vi "Main_PID.vi"() -> ()   [LabVIEW 2021]
doc: "This template is for the Queued Message Handler design pattern.\n\nThe Event Handling Loop generates messages based on user interface actions.\n\nThe Message Handling Loop processes messages generated by the Event Handling Loop, or by other messages. The messages are string values, so new messages can be added easily to the Message Cases case structure in the Message Handling Loop. Each message cluster can also provide an optional value for Message Data, which is a variant that can be converted to whatever message-specific data is required."
uses:
  Controls/UI Data.ctl
  support/Message Queue/Message Queue.lvlib
  support/User Event - Stop/User Event - Stop.lvlib
  support/Message Queue/Enqueue Message (Single).vi
  Controls/Status Lights.ctl
  Controls/Timer Actions.ctl
  <vilib>/ErrorRing/Error Ring.xnode
  <vilib>/Utility/error.llb/Error Cluster From Error Code.vi
panel:
  in  "Horizontal Slide Switch":bool
  out "Target Speed":dbl format="%.2f"
  in  "Target Pressure (Bar)":dbl
  in  "Start PID Control":bool
  out "Sampling Active":bool=TRUE
  out "Pressure":dbl(knob) scale=0.0..10.0
  out "Pressure (Bar)":dbl
  out "Sampling State":string
  in  "Start Pressure Logging":bool
  out "Speed Indicator":dbl
  in  "Release Brake":bool
  out "Status":T1
  in  "Speed (v)":dbl(knob) min=-5.0 max=5.0 scale=-5.0..5.0
  out "Status Message":string
  in  "Apply Brake":bool
  in  "Exit":bool
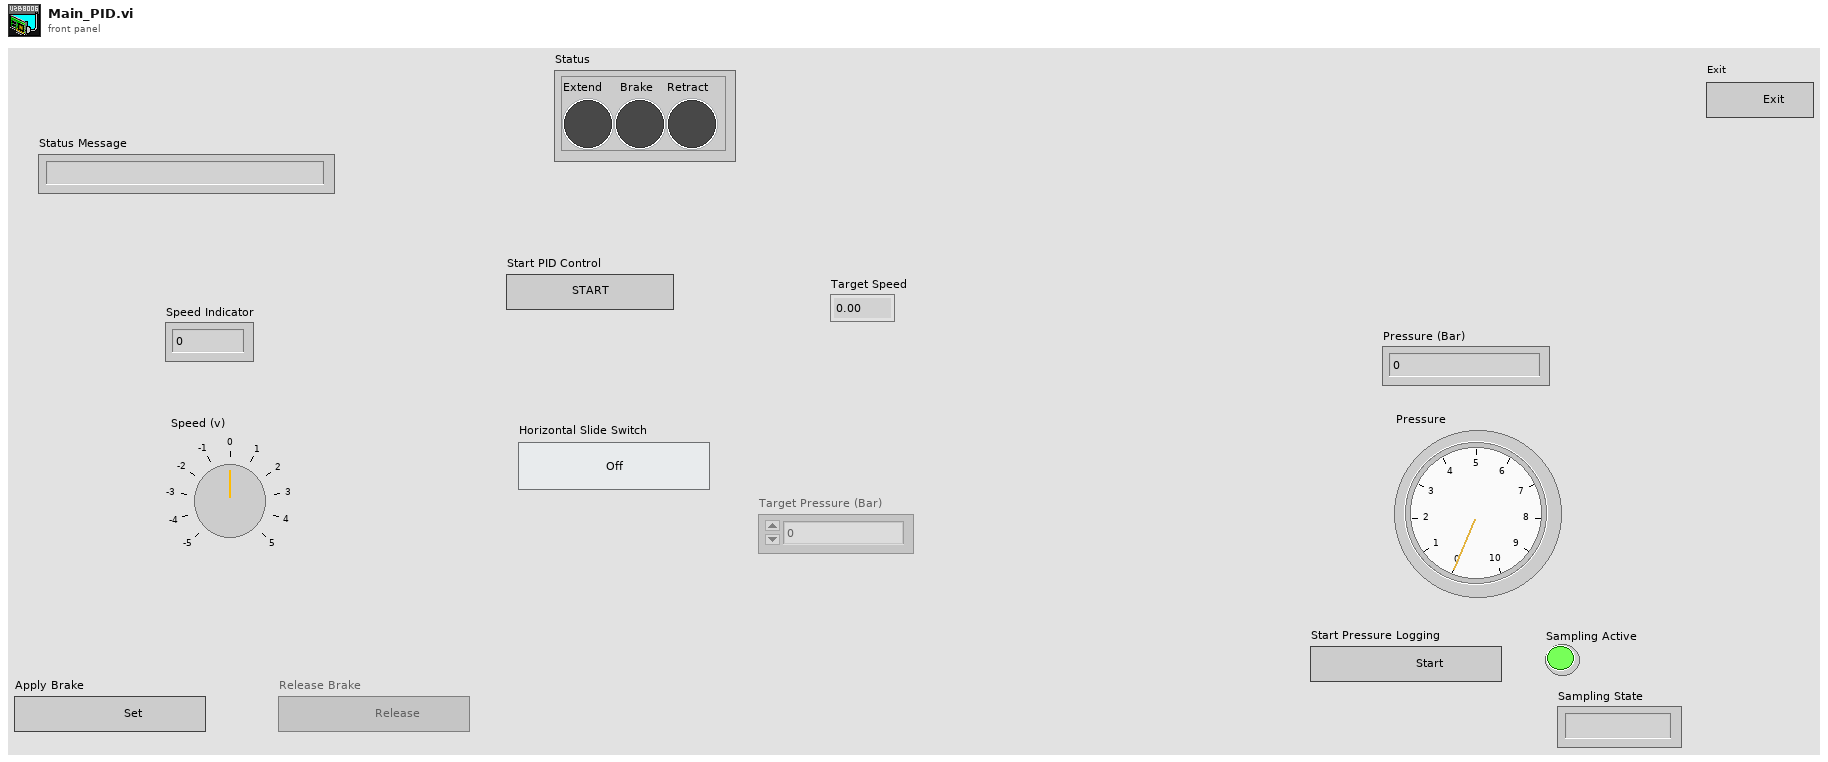
[diagram p1: front panel]
types:
  T1 = typedef "Status Lights.ctl" = cluster{"Extend":bool, "Brake":bool, "Retract":bool}
  T2 = cluster{"Apply Brake FP":enum8{"Enabled", "Disabled", "Disabled and Grayed Out"}, "Release Brake FP":enum8{"Enabled", "Disabled", "Disabled and Grayed Out"}, "Extend FP":enum8{"Enabled", "Disabled", "Disabled and Grayed Out"}, "Retract FP":enum8{"Enabled", "Disabled", "Disabled and Grayed Out"}, "Pressure Log FP":enum8{"Enabled", "Disabled", "Disabled and Grayed Out"}, "Speed FP":enum8{"Enabled", "Disabled", "Disabled and Grayed Out"}, "Target Pressure FP":enum8{"Enabled", "Disabled", "Disabled and Grayed Out"}}
  T3 = typedef "UI Data.ctl" = cluster{"Sampling State":string, "Status Message":string, "Speed":dbl, "Pressure":dbl, "Target Pressure":dbl, "Apply Brake Ref":refnum<vi>, "Release Brake Ref":refnum<vi>, "Extend Ref":refnum<vi>, "Retract Ref":refnum<vi>, "Pressure Ref":refnum<vi>, "Data Display Ref":refnum<vi>, "Exit Button Ref":refnum<vi>, "Speed Pressure Select":bool, "Status":T1}
  T4 = typedef "Message Queue.lvlib/All Message Queues.ctl" = cluster{"UI":refnum<queue>}
  T5 = typedef "DAQ Refnums.ctl" = cluster{"Direction Ref":refnum<k21>, "Brake Ref":refnum<k21>, "Speed Ref":refnum<k21>, "Pressure Ref":refnum<k21>}
  T6 = enum8{"Enabled", "Disabled", "Disabled and Grayed Out"}
  T7 = typedef "Timer Actions.ctl" = enum16{"Start Timer", "Restart Timer", "Check Timer", "Pause Timer", "Reset Timer", "Exit Timer"}
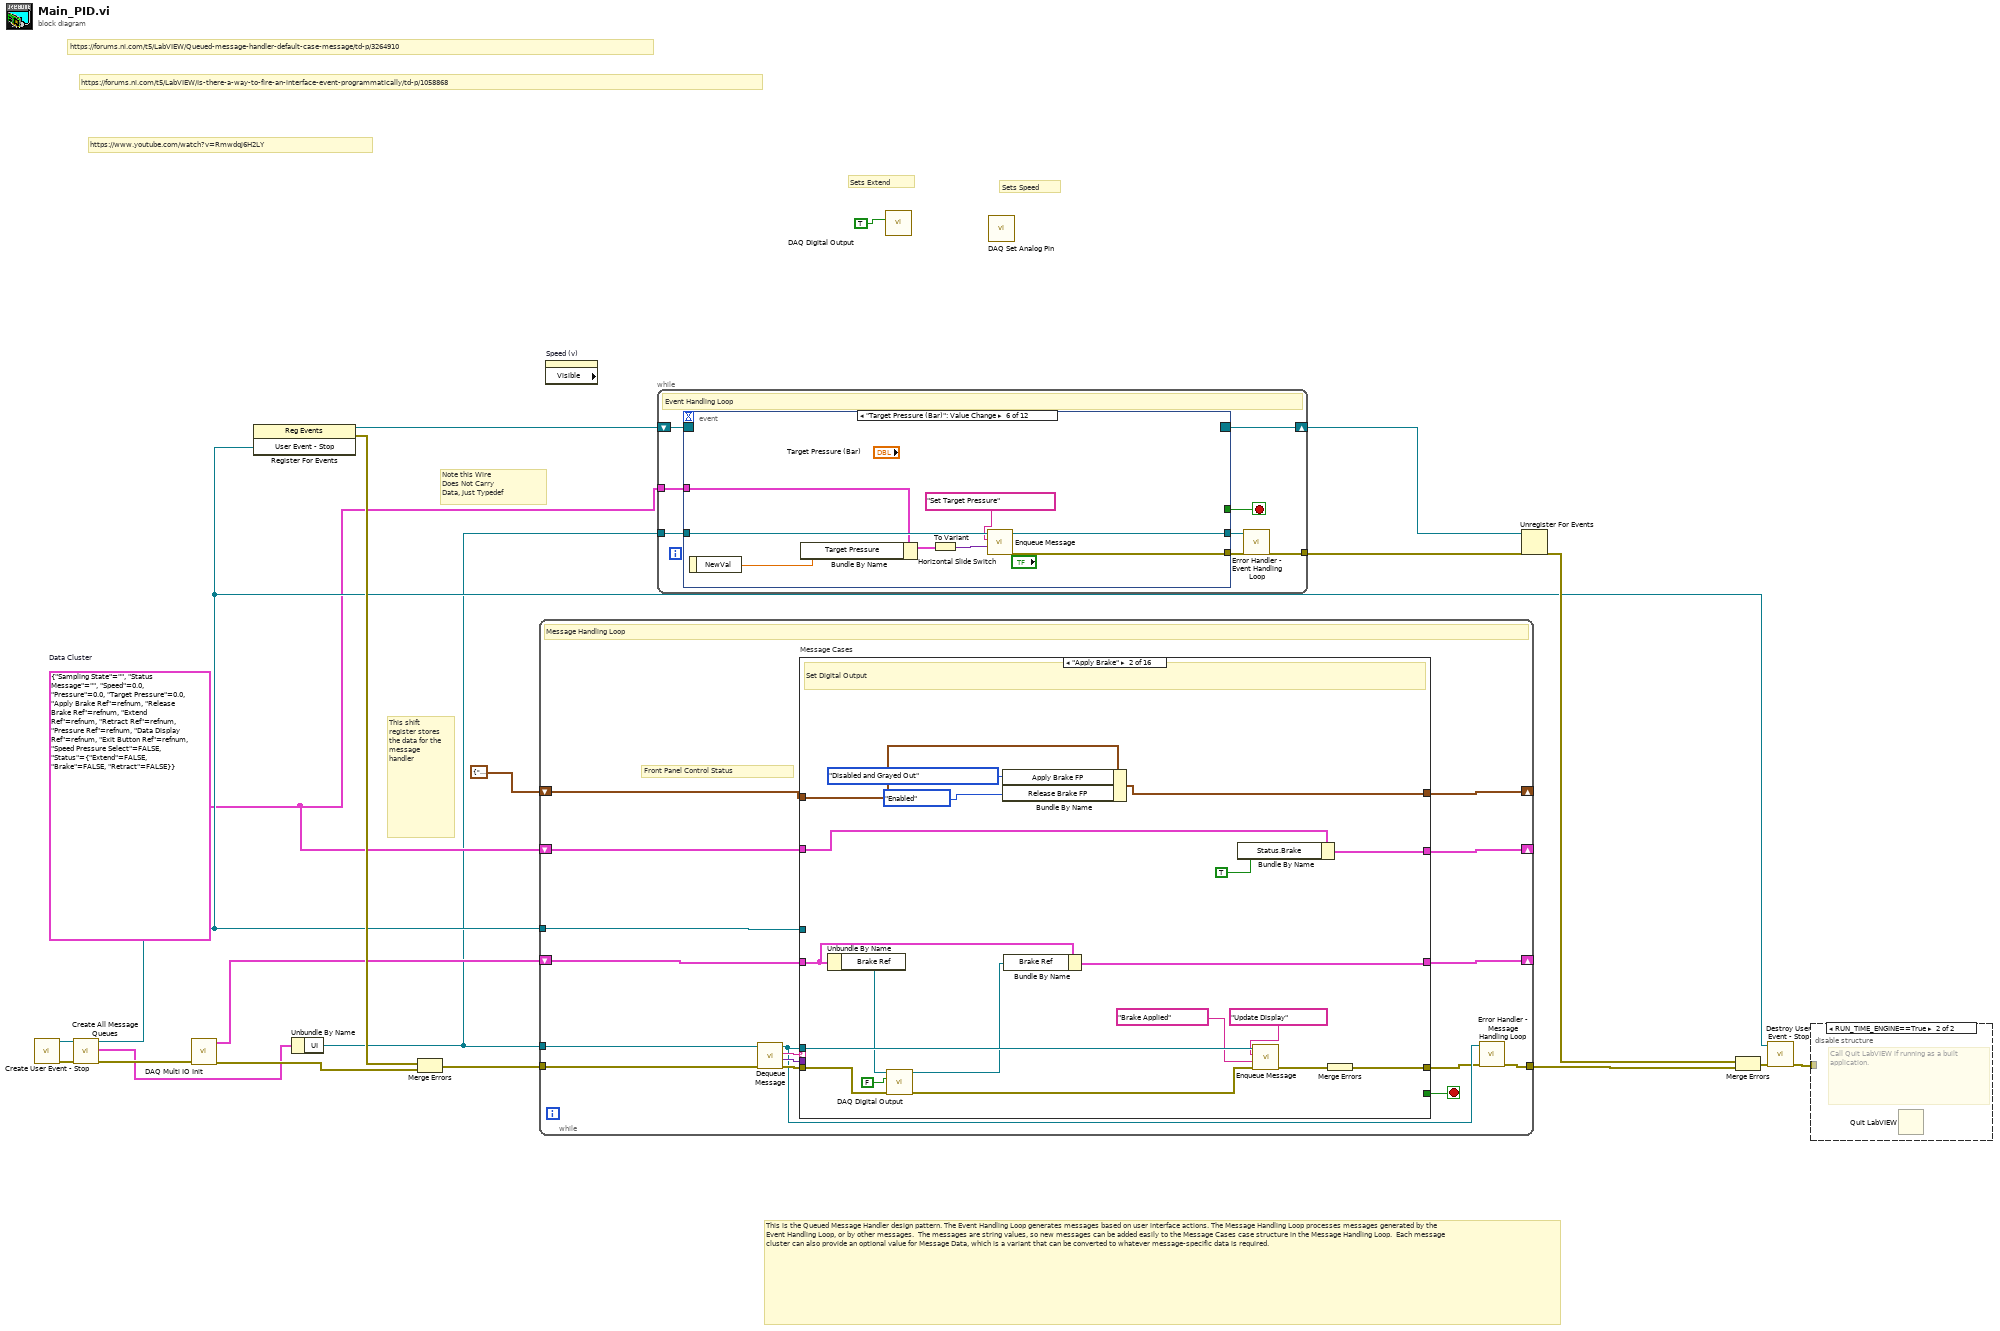
[diagram p0: block diagram]
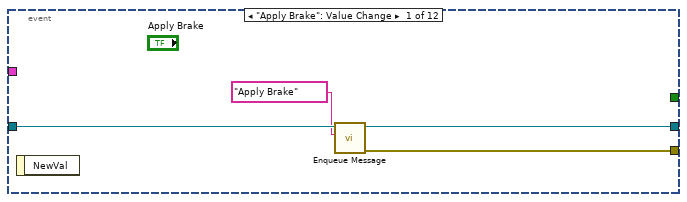
[diagram p3: hidden frame]
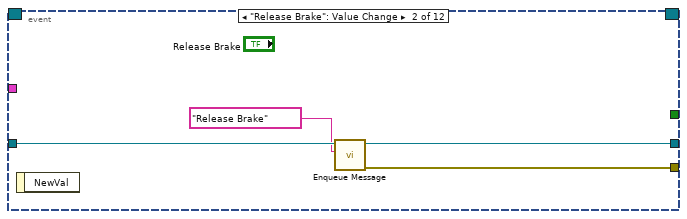
[diagram p4: hidden frame]
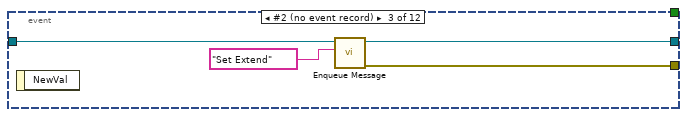
[diagram p5: hidden frame]
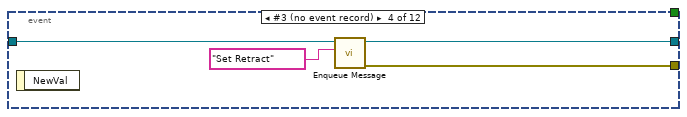
[diagram p6: hidden frame]
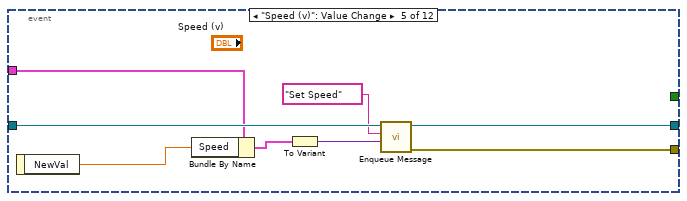
[diagram p7: hidden frame]
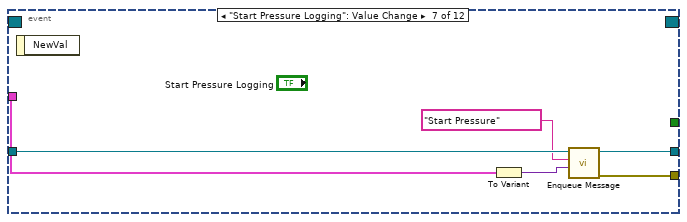
[diagram p8: hidden frame]
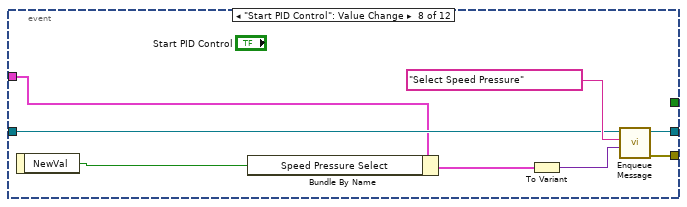
[diagram p9: hidden frame]
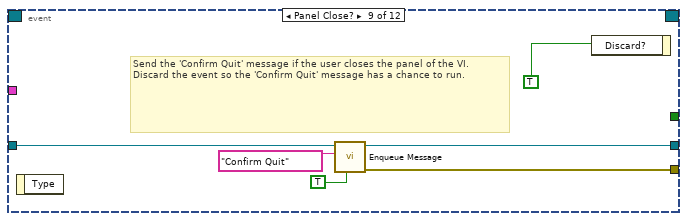
[diagram p10: hidden frame]
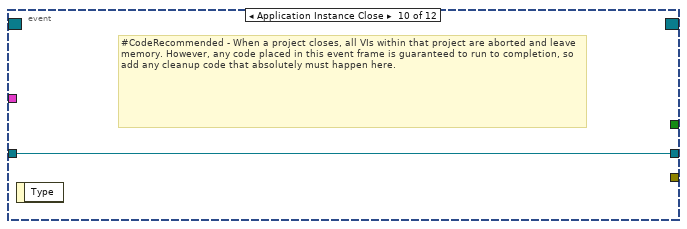
[diagram p11: hidden frame]
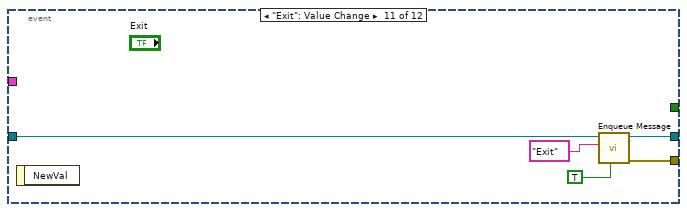
[diagram p12: hidden frame]
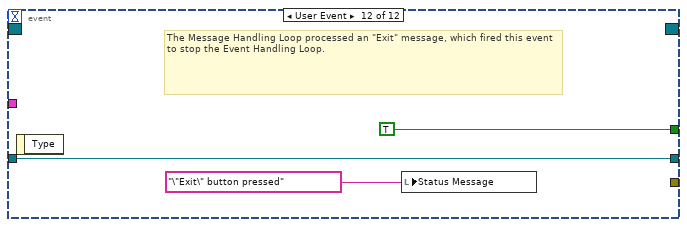
[diagram p13: hidden frame]
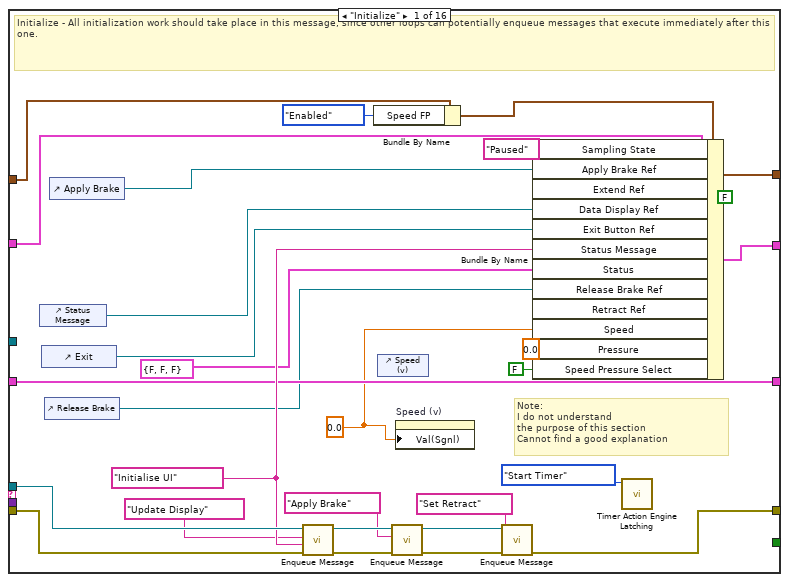
[diagram p14: hidden frame]
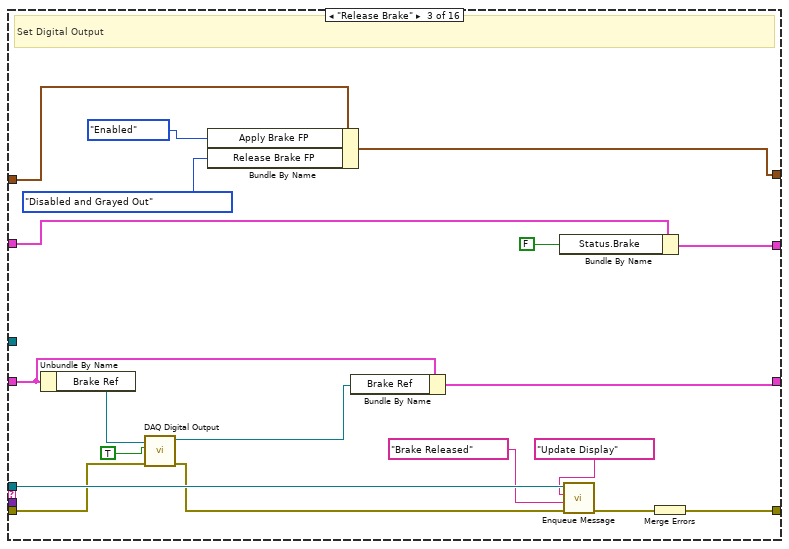
[diagram p15: hidden frame]
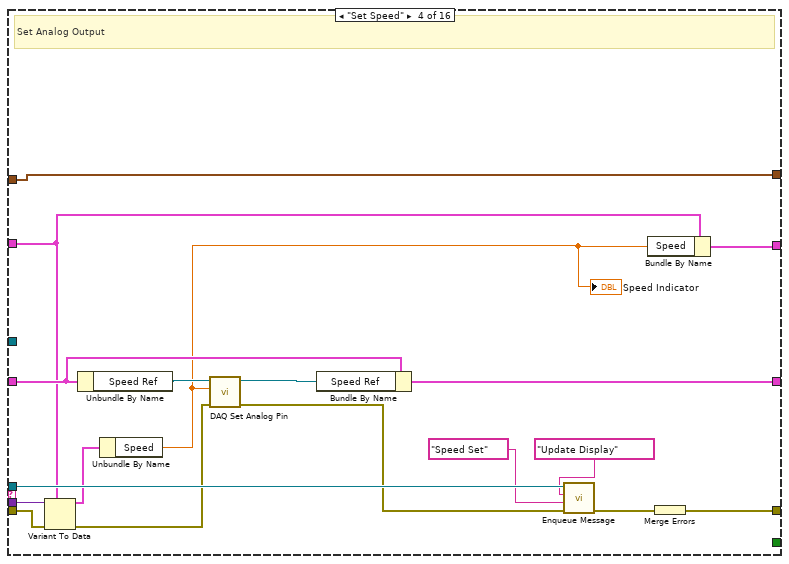
[diagram p16: hidden frame]
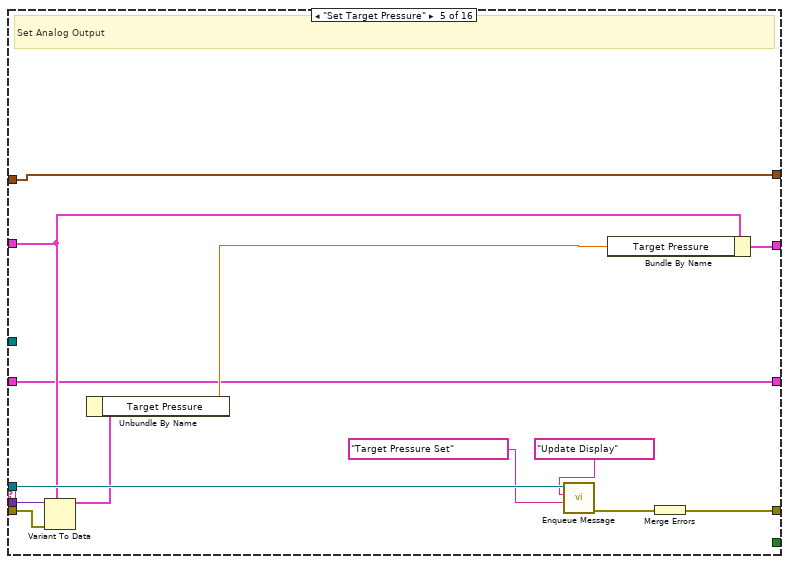
[diagram p17: hidden frame]
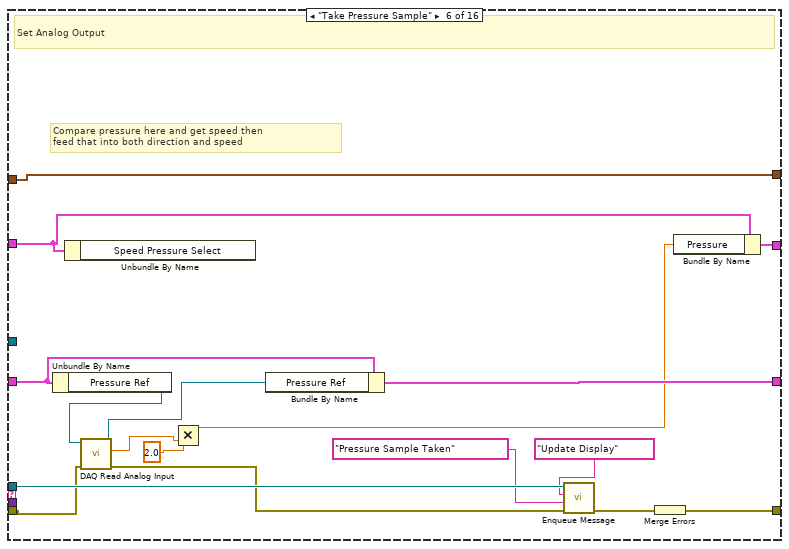
[diagram p18: hidden frame]
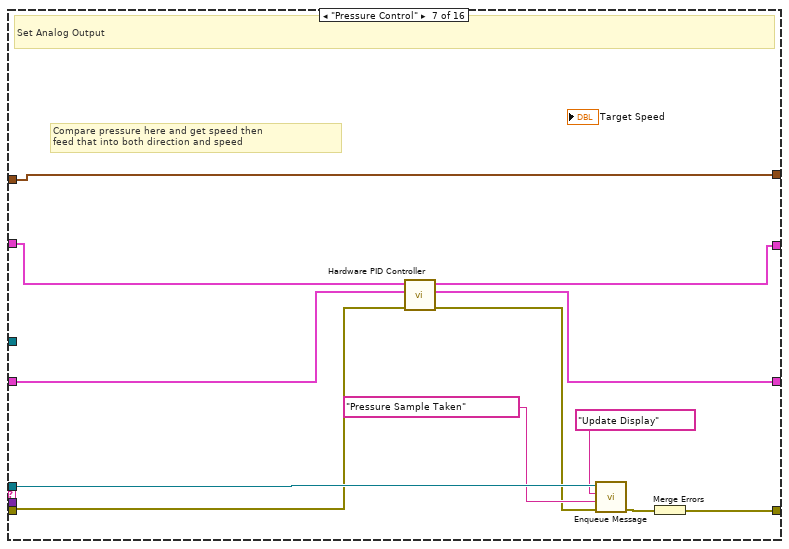
[diagram p19: hidden frame]
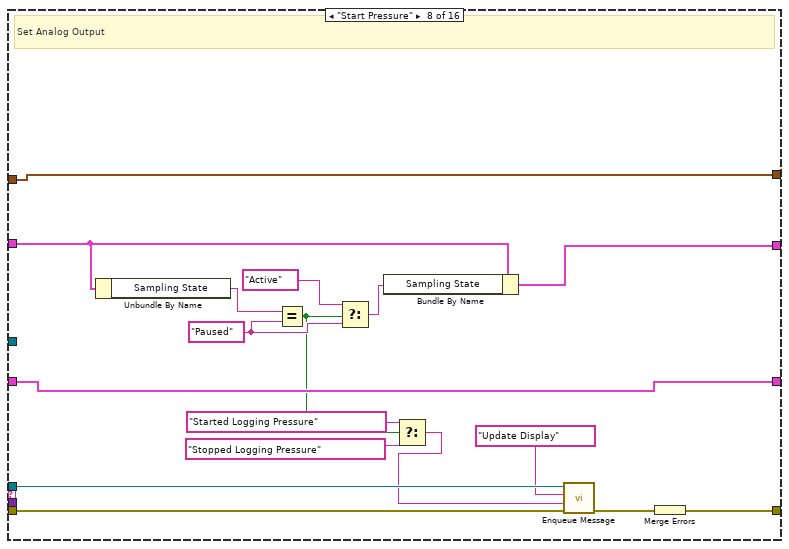
[diagram p20: hidden frame]
diagram:
  w4 = T3 {"Sampling State"="", "Status Message"="", "Speed"=0.0, "Pressure"=0.0, "Target Pressure"=0.0, "Apply Brake Ref"=refnum, "Release Brake Ref"=refnum, "Extend Ref"=refnum, "Retract Ref"=refnum, "Pressure Ref"=refnum, "Data Display Ref"=refnum, "Exit Button Ref"=refnum, "Speed Pressure Select"=FALSE, "Status"={"Extend"=FALSE, "Brake"=FALSE, "Retract"=FALSE}}  # Data Cluster
  # "Sets Speed"
  # "Sets Extend"
  # "Note this Wire\nDoes Not Carry\nData, Just Typedef"
  # "https://www.youtube.com/watch?v=Rmwdqj6H2LY"
  # "https://forums.ni.com/t5/LabVIEW/Is-there-a-way-to-fire-an-interface-event-programmatically/td-p/1058868"
  # "https://forums.ni.com/t5/LabVIEW/Queued-message-handler-default-case-message/td-p/3264910"
  # "This is the Queued Message Handler design pattern. The Event Handling Loop generates messages based on user interface actions. The Message Handling Loop processes messages generated by the Event Handling Loop, or by other messages.  The messages are string values, so new messages can be added easily to the Message Cases case structure in the Message Handling Loop.  Each message cluster can also provide an optional value for Message Data, which is a variant that can be converted to whatever message-specific data is required."
  # "This shift register stores the data for the message handler"
  n1 = call "Create User Event - Stop.vi"() -> ("error out"=w19:errorcluster, "User Event - Stop"=w8:refnum<user-event>)  [unwired: 10 in]
  n2 = call "Create All Message Queues.vi"("error in (no error)"=w19) -> ("error out"=w7:errorcluster, "Message Queues out"=w5:T4)  [unwired: 9 in]
  n3 = call "DAQ Multi IO Init.vi"("error in"=w7) -> ("error out"=w6:errorcluster, "DAQ Ref Cluster"=w9:T5)  [unwired: 9 in]
  n4 = register-events(w8) -> (reference out=w13:refnum<event-registration>, error out=w12:errorcluster)  [unwired: 2 in]
  n5 = Unbundle By Name(w5) -> ("UI"=w3:refnum<queue>)
  n6 = Merge Errors(w12, w6) -> (w10:errorcluster)
  n7 = while {
    tunnel: w3 -> [w29]
    shift-right: [w24] -> _
    shift-left: w4 -> [w35]
    tunnel: w8 -> [w33]
    tunnel: [w27] -> w11
    tunnel: w10 -> [w25]
    shift-right: [w22] -> _
    shift-left: w9 -> [w23]
    shift-right: [w20] -> _
    shift-left: T2 {"Apply Brake FP"=enum."Disabled and Grayed Out", "Release Brake FP"=enum."Disabled and Grayed Out", "Extend FP"=enum."Disabled and Grayed Out", "Retract FP"=enum."Disabled and Grayed Out", "Pressure Log FP"=enum."Disabled and Grayed Out", "Speed FP"=enum."Disabled and Grayed Out", "Target Pressure FP"=enum."Disabled and Grayed Out"} -> [w21]
    stop <- w34 stop-if-true
    # "Front Panel Control Status"
    # "Message Handling Loop"
    n8 = call "Dequeue Message.vi"("error in (no error)"=w25, "Message Queue"=w29) -> ("error out"=w32:errorcluster, "Message Data"=w30:variant, "Message"=w31:string, "dup Message Queue"=w28:refnum<queue>)  [unwired: 6 in]
    n9 = case "Message Cases" shown="\"Apply Brake\"" w31 {
      selector: w31 -> [_ _ _ _ _ _ _ _ _ _ _ _ _ _ _ w292]
      tunnel: w28 -> [w58 w79 w98 w116 w129 w146 w158 w175 w182 w205 _ w228 _ w243 w289 _]
      tunnel: w32 -> [w62 w77 w96 w107 w125 w135 w151 w167 w184 w209 w223 w232 w237 w247 w284 _]
      tunnel: [w45 w81 w100 w118 w131 w148 w160 w177 w183 w214 w217 w230 w235 w250 w286 w293] -> w26
      tunnel: w35 -> [w51 w71 w86 w104 w123 w133 w149 w168 w181 w197 w222 w231 w236 w241 w288 w294]
      tunnel: [w61 w74 w93 w103 w122 w141 w153 w170 w181 w197 w222 w231 w236 w240 w288 w294] -> w24
      tunnel: [_ _ _ _ _ _ _ _ _ _ _ _ _ _ TRUE _] -> w34
      tunnel: w30 -> [_ _ _ w108 w126 _ _ _ _ w210 w221 _ _ w248 w281 _]
      tunnel: w33 -> [_ _ _ _ _ _ _ _ _ _ _ _ _ _ w285 _]
      tunnel: w23 -> [w54 w69 w88 w113 w119 w143 w155 w171 w185 w212 w216 w225 w234 w249 w273 w291]
      tunnel: [w54 w68 w87 w112 w119 w142 w154 w171 w185 w212 w216 w225 w234 w249 w274 w291] -> w22
      tunnel: w21 -> [w38 w66 w85 w101 w120 w134 w150 w161 w178 w203 w215 w224 w233 w245 w267 w290]
      tunnel: [w39 w63 w82 w101 w120 w134 w150 w161 w178 w203 w215 w224 w233 w244 w267 w290] -> w20
      frame "Initialize" {
        (unwired) FALSE ("Clock Output")
        w52 = 0.0 ("Speed")
        w57 = "Initialise UI" ("Initial Message")
        # "Note:\nI do not understand\nthe purpose of this section\nCannot find a good explanation"
        # "Initialize - All initialization work should take place in this message, since other loops can potentially enqueue messages that execute immediately after this one."
        n10 = control-ref of="Status Message"() -> (w60:refnum<vi>)
        n11 = control-ref of="Exit"() -> (w59:refnum<vi>)
        n12 = control-ref of="Release Brake"() -> (w53:refnum<vi>)
        n13 = control-ref of="Apply Brake"() -> (w56:refnum<vi>)
        n14 = call-poly "Enqueue Message.vi"("error in (no error)"=w62, "Message Data"=w57, "Message"="Update Display", "Message Queue"=w58) -> ("error out"=w49:errorcluster, "dup Message Queue"=w48:refnum<queue>)  [unwired: 6 in]
        n15 = Bundle By Name(cluster=w38, "Speed FP"=T6."Enabled") -> (w39:T2)
        n16 = control-ref of="Speed (v)"() -> ()  [unwired: 1 out]
        n17 = call-poly "Enqueue Message.vi"("error in (no error)"=w49, "Message"="Apply Brake", "Message Queue"=w48) -> ("error out"=w46:errorcluster, "dup Message Queue"=w44:refnum<queue>)  [unwired: 7 in]
        n18 = property on="Speed (v)" class="Knob (strict)"("Val(Sgnl)"=w52) -> ()  [unwired: 2 in, 2 out]
        n19 = call-poly "Enqueue Message.vi"("error in (no error)"=w46, "Message"="Set Retract", "Message Queue"=w44) -> ("error out"=w45:errorcluster)  [unwired: 7 in, 1 out]
        n20 = Bundle By Name(cluster=w51, "Sampling State"="Paused", "Apply Brake Ref"=w56, "Data Display Ref"=w60, "Exit Button Ref"=w59, "Status Message"=w57, "Status"=T1 {"Extend"=FALSE, "Brake"=FALSE, "Retract"=FALSE}, "Release Brake Ref"=w53, "Speed"=w52, "Pressure"=0.0, "Speed Pressure Select"=FALSE) -> (w61:T3)  [unwired: 2 in]
        n21 = call "Timer Action Engine Latching.vi"("Action"=Timer_Actions."Start Timer") -> ()  [unwired: 7 in, 4 out]
      }
      frame "Apply Brake" {
        # "Set Digital Output"
        n22 = Unbundle By Name(w69) -> ("Brake Ref"=w70:refnum<k21>)
        n23 = call "DAQ Digital Output.vi"("error in"=w77, "data"=FALSE, "task/channels in"=w70) -> ("error out"=w76:errorcluster, "task out"=w67:refnum<k21>)  [unwired: 6 in, 1 out]
        n24 = Bundle By Name(cluster=w66, "Apply Brake FP"=T6."Disabled and Grayed Out" ("Disabled"), "Release Brake FP"=T6."Enabled" ("Disabled")) -> (w63:T2)
        n25 = Bundle By Name(cluster=w69, "Brake Ref"=w67) -> (w68:T5)
        n26 = Bundle By Name(cluster=w71, "Status.Brake"=TRUE) -> (w74:T3)
        n27 = call-poly "Enqueue Message.vi"("error in (no error)"=w76, "Message Data"="Brake Applied" ("\"Do Something\" button pressed"), "Message"="Update Display", "Message Queue"=w79) -> ("error out"=w80:errorcluster)  [unwired: 6 in, 1 out]
        n28 = Merge Errors(w80) -> (w81:errorcluster)
      }
      frame "Release Brake" {
        # "Set Digital Output"
        n29 = Unbundle By Name(w88) -> ("Brake Ref"=w90:refnum<k21>)
        n30 = call "DAQ Digital Output.vi"("error in"=w96, "data"=TRUE, "task/channels in"=w90) -> ("error out"=w95:errorcluster, "task out"=w89:refnum<k21>)  [unwired: 6 in, 1 out]
        n31 = Bundle By Name(cluster=w85, "Apply Brake FP"=T6."Enabled" ("Disabled"), "Release Brake FP"=T6."Disabled and Grayed Out" ("Disabled")) -> (w82:T2)
        n32 = Bundle By Name(cluster=w88, "Brake Ref"=w89) -> (w87:T5)
        n33 = Bundle By Name(cluster=w86, "Status.Brake"=FALSE ("Boolean")) -> (w93:T3)
        n34 = call-poly "Enqueue Message.vi"("error in (no error)"=w95, "Message Data"="Brake Released" ("\"Do Something\" button pressed"), "Message"="Update Display", "Message Queue"=w98) -> ("error out"=w99:errorcluster)  [unwired: 6 in, 1 out]
        n35 = Merge Errors(w99) -> (w100:errorcluster)
      }
      frame "Set Speed" {
        # "Set Analog Output"
        n36 = Variant To Data(error in=w107, type=w104, Variant=w108) -> (data=w105:T3, error out=w106:errorcluster)
        n37 = Unbundle By Name(w113) -> ("Speed Ref"=w111:refnum<k21>)
        n38 = Unbundle By Name(w105) -> ("Speed"=w102:dbl)
        "Speed Indicator" <- w102
        n39 = call "DAQ Set Analog Pin.vi"("error in"=w106, "Voltage"=w102, "task/channels in"=w111) -> ("error out"=w109:errorcluster, "task out"=w110:refnum<k21>)  [unwired: 6 in, 1 out]
        n40 = Bundle By Name(cluster=w113, "Speed Ref"=w110) -> (w112:T5)
        n41 = call-poly "Enqueue Message.vi"("error in (no error)"=w109, "Message Data"="Speed Set" ("\"Do Something\" button pressed"), "Message"="Update Display", "Message Queue"=w116) -> ("error out"=w117:errorcluster)  [unwired: 6 in, 1 out]
        n42 = Bundle By Name(cluster=w104, "Speed"=w102) -> (w103:T3)
        n43 = Merge Errors(w117) -> (w118:errorcluster)
      }
      frame "Set Target Pressure" {
        # "Set Analog Output"
        n44 = Variant To Data(error in=w125, type=w123, Variant=w126) -> (data=w124:T3)  [unwired: 1 out]
        n45 = Unbundle By Name(w124) -> ("Target Pressure"=w121:dbl)
        n46 = call-poly "Enqueue Message.vi"("Message Data"="Target Pressure Set" ("\"Do Something\" button pressed"), "Message"="Update Display", "Message Queue"=w129) -> ("error out"=w130:errorcluster)  [unwired: 7 in, 1 out]
        n47 = Bundle By Name(cluster=w123, "Target Pressure"=w121) -> (w122:T3)
        n48 = Merge Errors(w130) -> (w131:errorcluster)
      }
      frame "Take Pressure Sample" {
        # "Compare pressure here and get speed then \nfeed that into both direction and speed"
        # "Set Analog Output"
        n49 = Unbundle By Name(w143) -> ("Pressure Ref"=w140:refnum<k21>)
        n50 = Unbundle By Name(w133) -> ()  [unwired: 1 out]
        n51 = call "DAQ Read Analog Input.vi"("error in"=w135, "task/channels in"=w140) -> ("error out"=w139:errorcluster, "Voltage"=w137:dbl, "task out"=w138:refnum<k21>)  [unwired: 7 in]
        n52 = Multiply(x=2.0, y=w137) -> (x*y=w132:dbl)
        n53 = Bundle By Name(cluster=w143, "Pressure Ref"=w138) -> (w142:T5)
        n54 = call-poly "Enqueue Message.vi"("error in (no error)"=w139, "Message Data"="Pressure Sample Taken" ("\"Do Something\" button pressed"), "Message"="Update Display", "Message Queue"=w146) -> ("error out"=w147:errorcluster)  [unwired: 6 in, 1 out]
        n55 = Merge Errors(w147) -> (w148:errorcluster)
        n56 = Bundle By Name(cluster=w133, "Pressure"=w132) -> (w141:T3)
      }
      frame "Pressure Control" {
        # "Compare pressure here and get speed then \nfeed that into both direction and speed"
        # "Set Analog Output"
        n57 = call "Hardware PID Controller.vi"("error in (no error)"=w151, "DAQ Ref Cluster in"=w155, "State Machine Data"=w149) -> ("error out"=w152:errorcluster, "DAQ Ref Cluster out"=w154:T5, "Data Cluster out"=w153:T3)  [unwired: 6 in]
        n58 = call-poly "Enqueue Message.vi"("error in (no error)"=w152, "Message Data"="Pressure Sample Taken" ("\"Do Something\" button pressed"), "Message"="Update Display", "Message Queue"=w158) -> ("error out"=w159:errorcluster)  [unwired: 6 in, 1 out]
        n59 = Merge Errors(w159) -> (w160:errorcluster)
      }
      frame "Start Pressure" {
        w165 = "Paused" ("y")
        # "Set Analog Output"
        n60 = Unbundle By Name(w168) -> ("Sampling State"=w166:string)
        n61 = Equal?(x=w166, y=w165) -> (x = y?=w162:bool)
        n62 = Select(t="Active", s=w162, f=w165) -> (s? t:f=w163:string)
        n63 = Bundle By Name(cluster=w168, "Sampling State"=w163) -> (w170:T3)
        n64 = Select(t="Started Logging Pressure" ("Status Message"), s=w162, f="Stopped Logging Pressure") -> (s? t:f=w169:string)
        n65 = call-poly "Enqueue Message.vi"("error in (no error)"=w167, "Message Data"=w169, "Message"="Update Display", "Message Queue"=w175) -> ("error out"=w176:errorcluster)  [unwired: 6 in, 1 out]
        n66 = Merge Errors(w176) -> (w177:errorcluster)
      }
      frame "Wait" {
        # "Wait case - wait for user input Or Timing Trigger"
        n67 = Unbundle By Name(w181) -> ("Sampling State"=w180:string)
        n68 = case shown="\"Paused\", Default" w180 {
          tunnel: [FALSE ("Sampling Active") TRUE ("Sampling Active")] -> w179
          frame "Paused", Default {
          }
          frame "Active" {
          }
        }
        "Sampling Active" <- w179
        n69 = case shown="True" w179 {
          selector: w179 -> [w188 _]
          tunnel: w184 -> [w189 w194]
          tunnel: [w189 w193] -> w183
          tunnel: w182 -> [_ w192]
          tunnel: [w188 TRUE] -> _
          frame False {
          }
          frame True {
            n70 = call-poly "Enqueue Message.vi"("error in (no error)"=w194, "Message"="Take Pressure Sample", "Message Queue"=w192) -> ("error out"=w193:errorcluster)  [unwired: 7 in, 1 out]
          }
        }
      }
      frame "Update Display" {
        # "Update Display - Convert the message data to a string to display in the Data Display indicator."
        n71 = Unbundle By Name(w203) -> ("Apply Brake FP"=w202:T6, "Release Brake FP"=w201:T6, "Pressure Log FP"=w200:T6, "Speed FP"=w199:T6, "Target Pressure FP"=w198:T6)  [unwired: 2 out]
        n72 = Unbundle By Name(w197) -> ("Status"=→"Status":T1, "Sampling State"=→"Sampling State":string, "Pressure"=→"Pressure (Bar)" →"Pressure":dbl)
        n73 = Variant To Data(error in=w209, type="" ("Status Message"), Variant=w210) -> (data=→"Status Message":string, error out=w207:errorcluster)
        n74 = property on="Start Pressure Logging" class="Bool"("DisabledEnum"=w200) -> ()  [unwired: 2 in, 2 out]
        n75 = property on="Apply Brake" class="Bool"("DisabledEnum"=w202) -> ()  [unwired: 2 in, 2 out]
        n76 = property on="Speed (v)" class="Knob (strict)"("DisabledEnum"=w199) -> ()  [unwired: 2 in, 2 out]
        n77 = property on="Release Brake" class="Bool"("DisabledEnum"=w201) -> ()  [unwired: 2 in, 2 out]
        n78 = property on="Target Pressure (Bar)" class="DigNum (strict)"("DisabledEnum"=w198) -> ()  [unwired: 2 in, 2 out]
        n79 = call-poly "Enqueue Message.vi"("error in (no error)"=w207, "Message"="Wait", "Message Queue"=w205) -> ("error out"=w206:errorcluster)  [unwired: 7 in, 1 out]
        n80 = Merge Errors(w206) -> (w214:errorcluster)
      }
      frame "Error" {
        # "#CodeRecommended - If you ever change the name of this \"Error\" message, you'll need to update the name in the Check Loop Error.vi as well."
        # "#CodeRecommended - Consider creating a system for logging errors in some way. These errors are for notification purposes only. Handling of specific errors should be performed in the message frames that generated the error."
        # "Error - Display an error dialog. This message is sent by the \"Error Handler\" VIs at the end of other loops in this application."
        n81 = Variant To Data(error in=w223, type=errorcluster {"status"=FALSE, "code"=0, "source"=""} ("error constant"), Variant=w221) -> (data=w219:errorcluster, error out=w218:errorcluster)
        n82 = call <vilib>:"Simple Error Handler.vi"("error in (no error)"=w219) -> ()  [unwired: 4 in, 5 out]
        n83 = Merge Errors(w218) -> (w217:errorcluster)
      }
      frame "Confirm Quit" {
        # "#CodeNeeded - If you want to provide an \"Are you sure\" dialog (or some other notification) before the application exits, place that code here. This message is typically sent from a Panel Close? event."
        # "Confirm Quit - Message that can confirm whether or not the user wants to exit the application."
        n84 = call-poly "Enqueue Message.vi"("Priority Message? (F)"=TRUE, "error in (no error)"=w232, "Message"="Exit", "Message Queue"=w228) -> ("error out"=w229:errorcluster)  [unwired: 6 in, 1 out]
        n85 = Merge Errors(w229) -> (w230:errorcluster)
      }
      frame "---Copy This Frame---" {
        # "Duplicate this frame when creating new messages.  Change this comment in the duplicated frame to describe this message."
        n86 = Merge Errors(w237) -> (w235:errorcluster)
      }
      frame "Select Speed Pressure" {
        # "Duplicate this frame when creating new messages.  Change this comment in the duplicated frame to describe this message."
        n87 = Variant To Data(error in=w247, type=w241, Variant=w248) -> (data=w240:T3, error out=w246:errorcluster)
        n88 = Unbundle By Name(w240) -> ("Speed Pressure Select"=w239:bool)
        n89 = case shown="False" w239 {
          tunnel: w245 -> [w258 w266]
          tunnel: [w257 w265] -> w244
          tunnel: ["Changing Control Mode: Pressure" ("Message") "Changing Control Mode: Pressure" ("Message")] -> w238
          frame True {
            n90 = Bundle By Name(cluster=w258, "Target Pressure FP"=T6."Enabled", "Pressure Log FP"=T6."Disabled and Grayed Out", "Speed FP"=T6."Disabled and Grayed Out", "Extend FP"=T6."Disabled and Grayed Out", "Retract FP"=T6."Disabled and Grayed Out") -> (w257:T2)
          }
          frame False {
            n91 = Bundle By Name(cluster=w266, "Target Pressure FP"=T6."Disabled and Grayed Out", "Pressure Log FP"=T6."Enabled", "Speed FP"=T6."Enabled", "Extend FP"=T6."Disabled and Grayed Out", "Retract FP"=T6."Enabled") -> (w265:T2)
          }
        }
        n92 = call-poly "Enqueue Message.vi"("Message Data"=w238, "Message"="Update Display", "Message Queue"=w243) -> ()  [unwired: 7 in, 2 out]
        n93 = Merge Errors(w246) -> (w250:errorcluster)
      }
      frame "Exit" {
        # "Stop the VI"
        # "Release the message queue reference"
        # "Exit - Exit the application."
        n94 = Release Queue(queue=w289, error in (no error)=w284) -> (error out=w280:errorcluster)  [unwired: 1 in, 2 out]
        n95 = call "Fire User Event - Stop.vi"("User Event - Stop"=w285) -> ("error out"=w269:errorcluster)  [unwired: 10 in]
        n96 = Variant To Data(type=errorcluster {"status"=FALSE, "code"=0, "source"=""} ("error constant"), Variant=w281) -> (data=w282:errorcluster)  [unwired: 1 in, 1 out]
        n97 = Unbundle By Name(w273) -> ("Direction Ref"=w277:refnum<k21>, "Brake Ref"=w276:refnum<k21>, "Speed Ref"=w275:refnum<k21>)  [unwired: 1 out]
        n98 = call <vilib>:"Simple Error Handler.vi"("error in (no error)"=w282) -> ()  [unwired: 4 in, 5 out]
        n99 = call <vilib>:"DAQmx Clear Task.vi"("task in"=w275, "error in"=w280) -> ("error out"=w279:errorcluster)  [unwired: 13 in]
        n100 = call <vilib>:"DAQmx Clear Task.vi"("task in"=w276, "error in"=w279) -> ("error out"=w278:errorcluster)  [unwired: 13 in]
        n101 = call <vilib>:"DAQmx Clear Task.vi"("task in"=w277, "error in"=w278) -> ("error out"=w268:errorcluster)  [unwired: 13 in]
        n102 = Bundle By Name(cluster=w273, "Direction Ref"=refnum<k21> refnum, "Brake Ref"=refnum<k21> refnum, "Speed Ref"=refnum<k21> refnum) -> (w274:T5)  [unwired: 1 in]
        n103 = Merge Errors(w269, w268) -> (w286:errorcluster)
      }
      frame Default {
        # "'Default' case only runs if there is a message that isn't defined in any of the other cases.  Output a programming error."
        n104 = xnode "Error Ring"("parameter 0"=w292) -> ("error out"=w293:errorcluster)
      }
    }
    n105 = call "Error Handler - Message Handling Loop.vi"("error in (no error)"=w26, "Message Queue"=w28) -> ("dup error in"=w27:errorcluster)  [unwired: 8 in, 1 out]
  }
  n106 = property on="Speed (v)" class="Knob (strict)" props=["Visible"]() -> ()  [unwired: 2 in, 3 out]
  n107 = while {
    tunnel: w3 -> [w309]
    shift-right: [w307] -> w16
    shift-left: w13 -> [w308]
    tunnel: [w303] -> w14
    tunnel: w4 -> [w302]
    stop <- w305 stop-if-true
    # "Event Handling Loop"
    n108 = event shown="[5] \"Target Pressure (Bar)\": Value Change" {
      selector: w308 -> [_ _ _ _ _ _ _ _ _ _ _ _]
      dyn-events: [_ _ _ _ _ _ _ _ _ _ _ _] -> w307
      timeout: _ -> [_ _ _ _ _ _ _ _ _ _ _ _]
      tunnel: [_ _ _ _ _ _ _ _ _ _ _ TRUE ("Discard?")] -> w305
      tunnel: w309 -> [w313 w317 w321 w325 w333 w341 w345 w354 w360 w362 w367 w370]
      tunnel: [w310 w314 w318 w322 w330 w338 w346 w352 w359 _ w366 _] -> w306
      tunnel: [w312 w316 w320 w324 w332 w340 w347 w353 w358 w362 w365 w370] -> w304
      tunnel: w302 -> [_ _ _ _ w326 w334 w342 w351 _ _ _ _]
      event "Apply Brake": Value Change {
        n109 = event-data() -> ()  [unwired: 1 in, 1 out]
        n110 = call-poly "Enqueue Message.vi"("Message"="Apply Brake", "Message Queue"=w313) -> ("error out"=w310:errorcluster, "dup Message Queue"=w312:refnum<queue>)  [unwired: 8 in]
      }
      event "Release Brake": Value Change {
        n111 = event-data() -> ()  [unwired: 1 in, 1 out]
        n112 = call-poly "Enqueue Message.vi"("Message"="Release Brake", "Message Queue"=w317) -> ("error out"=w314:errorcluster, "dup Message Queue"=w316:refnum<queue>)  [unwired: 8 in]
      }
      event #2 (no event record) {
        n113 = event-data() -> ()  [unwired: 1 in, 1 out]
        n114 = call-poly "Enqueue Message.vi"("Message"="Set Extend", "Message Queue"=w321) -> ("error out"=w318:errorcluster, "dup Message Queue"=w320:refnum<queue>)  [unwired: 8 in]
      }
      event #3 (no event record) {
        n115 = event-data() -> ()  [unwired: 1 in, 1 out]
        n116 = call-poly "Enqueue Message.vi"("Message"="Set Retract", "Message Queue"=w325) -> ("error out"=w322:errorcluster, "dup Message Queue"=w324:refnum<queue>)  [unwired: 8 in]
      }
      event "Speed (v)": Value Change {
        n117 = event-data() -> ("NewVal"=w328:dbl)  [unwired: 1 in]
        n118 = Bundle By Name(cluster=w326, "Speed"=w328) -> (w327:T3)
        n119 = To Variant(anything=w327) -> (Variant=w329:variant)
        n120 = call-poly "Enqueue Message.vi"("Message Data"=w329, "Message"="Set Speed", "Message Queue"=w333) -> ("error out"=w330:errorcluster, "dup Message Queue"=w332:refnum<queue>)  [unwired: 7 in]
      }
      event "Target Pressure (Bar)": Value Change {
        n121 = event-data() -> ("NewVal"=w336:dbl)  [unwired: 1 in]
        n122 = Bundle By Name(cluster=w334, "Target Pressure"=w336) -> (w335:T3)
        n123 = To Variant(anything=w335) -> (Variant=w337:variant)
        n124 = call-poly "Enqueue Message.vi"("Message Data"=w337, "Message"="Set Target Pressure", "Message Queue"=w341) -> ("error out"=w338:errorcluster, "dup Message Queue"=w340:refnum<queue>)  [unwired: 7 in]
      }
      event "Start Pressure Logging": Value Change {
        n125 = event-data() -> ()  [unwired: 1 in, 1 out]
        n126 = To Variant(anything=w342) -> (Variant=w343:variant)
        n127 = call-poly "Enqueue Message.vi"("Message Data"=w343, "Message"="Start Pressure", "Message Queue"=w345) -> ("error out"=w346:errorcluster, "dup Message Queue"=w347:refnum<queue>)  [unwired: 7 in]
      }
      event "Start PID Control": Value Change {
        n128 = event-data() -> ("NewVal"=w348:bool)  [unwired: 1 in]
        n129 = Bundle By Name(cluster=w351, "Speed Pressure Select"=w348) -> (w350:T3)
        n130 = To Variant(anything=w350) -> (Variant=w349:variant)
        n131 = call-poly "Enqueue Message.vi"("Message Data"=w349, "Message"="Select Speed Pressure", "Message Queue"=w354) -> ("error out"=w352:errorcluster, "dup Message Queue"=w353:refnum<queue>)  [unwired: 7 in]
      }
      event Panel Close? {
        # "Send the 'Confirm Quit' message if the user closes the panel of the VI. Discard the event so the 'Confirm Quit' message has a chance to run."
        n132 = event-data() -> ()  [unwired: 1 in, 1 out]
        n133 = call-poly "Enqueue Message.vi"("Priority Message? (F)"=TRUE, "Message"="Confirm Quit", "Message Queue"=w360) -> ("error out"=w359:errorcluster, "dup Message Queue"=w358:refnum<queue>)  [unwired: 7 in]
        n134 = event-data("Discard?"=TRUE) -> ()  [unwired: 1 in, 1 out]
      }
      event Application Instance Close {
        # "#CodeRecommended - When a project closes, all VIs within that project are aborted and leave memory. However, any code placed in this event frame is guaranteed to run to completion, so add any cleanup code that absolutely must happen here."
        n135 = event-data() -> ()  [unwired: 1 in, 1 out]
      }
      event "Exit": Value Change {
        n136 = event-data() -> ()  [unwired: 1 in, 1 out]
        n137 = call-poly "Enqueue Message.vi"("Priority Message? (F)"=TRUE, "Message"="Exit", "Message Queue"=w367) -> ("error out"=w366:errorcluster, "dup Message Queue"=w365:refnum<queue>)  [unwired: 7 in]
      }
      event User Event {
        # "The Message Handling Loop processed an \"Exit\" message, which fired this event to stop the Event Handling Loop."
        n138 = event-data() -> ()  [unwired: 1 in, 1 out]
        n139 = local write "Status Message"("\"Exit\" button pressed" ("VI Stopped")) -> ()
      }
    }
    n140 = call "Error Handler - Event Handling Loop.vi"("error in (no error)"=w306, "Message Queue"=w304) -> ("dup error in"=w303:errorcluster)  [unwired: 8 in, 1 out]
  }
  n141 = call "DAQ Digital Output.vi"("data"=TRUE) -> ()  [unwired: 8 in, 3 out]
  n142 = call "DAQ Set Analog Pin.vi"() -> ()  [unwired: 9 in, 3 out]
  n143 = Unregister For Events(event registration refnum=w16, error in=w14) -> (error out=w17:errorcluster)
  n144 = Merge Errors(w17, w11) -> (w18:errorcluster)
  n145 = call "Destroy User Event - Stop.vi"("error in (no error)"=w18, "User Event - Stop"=w8) -> ("error out"=w15:errorcluster)  [unwired: 9 in]
  n146 = disable-structure shown="RUN_TIME_ENGINE==True" {
    disable-tunnel: w15 -> [_ _]
    frame condition #0 (active) {
    }
    frame condition #1 {
      # "Call Quit LabVIEW if running as a built application."
      n147 = Quit LabVIEW() -> ()  [unwired: 1 in]
    }
  }
